vi "Untitled 4 (SubVI).vi"(10 "ID Query":string, 11 "VISA Refnum in":refnum<visa-resource-name>) -> (3 "read buffer":string)   [LabVIEW 2020]
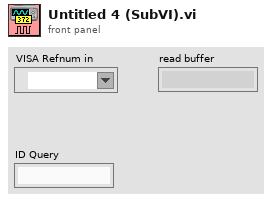
[diagram p1: front panel]
types:
  T1 = cluster{"Baud Rate":u32, "Parity":u16, "Data Bits":u16, "Stop Bits":u16, "Flow Control":u16}
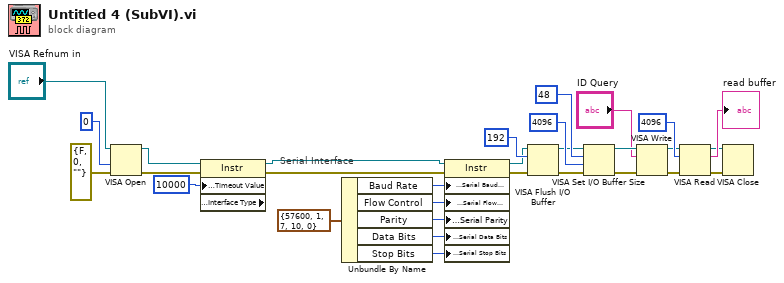
[diagram p0: block diagram]
diagram:
  # "Serial Interface"
  n1 = VISA Open(access mode=u32 0, error in (no error)=errorcluster {"status"=FALSE, "code"=0, "source"=""}, VISA resource name="VISA Refnum in") -> (VISA resource name=w5:refnum<visa-resource-name>, error out=w6:errorcluster)  [unwired: 2 in]
  n2 = property class="Instr" props=["General Settings:Timeout Value", "Interface Information:Interface Type"](reference=w5, error in=w6, "General Settings:Timeout Value"=u32 10000) -> (reference out=w7:refnum<visa-resource-name>, error out=w8:errorcluster)  [unwired: 1 out]
  n3 = Unbundle By Name(T1 {"Baud Rate"=57600, "Parity"=1, "Data Bits"=7, "Stop Bits"=10, "Flow Control"=0} ("Serial Configuration")) -> ("Baud Rate"=w20:u32, "Flow Control"=w24:u16, "Parity"=w22:u16, "Data Bits"=w21:u16, "Stop Bits"=w25:u16)
  n4 = property class="Instr"(reference=w7, error in=w8, "Serial Settings:Serial Baud Rate"=w20, "Serial Settings:Serial Flow Control"=w24, "Serial Settings:Serial Parity"=w22, "Serial Settings:Serial Data Bits"=w21, "Serial Settings:Serial Stop Bits"=w25) -> (reference out=w19:refnum<visa-resource-name>, error out=w17:errorcluster)
  n5 = VISA Flush I/O Buffer(VISA resource name=w19, mask (16)=u16 192, error in (no error)=w17) -> (VISA resource name out=w16:refnum<visa-resource-name>, error out=w18:errorcluster)
  n6 = VISA Set I/O Buffer Size(VISA resource name=w16, mask (16)=u16 48, size (4096)=u32 4096 ("size (0)"), error in (no error)=w18) -> (VISA resource name out=w30:refnum<visa-resource-name>, error out=w29:errorcluster)
  n7 = VISA Write(VISA resource name=w30, write buffer="ID Query", error in (no error)=w29) -> (VISA resource name out=w12:refnum<visa-resource-name>, error out=w11:errorcluster)  [unwired: 1 out]
  n8 = VISA Read(VISA resource name=w12, byte count=u32 4096, error in (no error)=w11) -> (VISA resource name out=w2:refnum<visa-resource-name>, read buffer=→"read buffer":string, error out=w1:errorcluster)  [unwired: 1 out]
  n9 = VISA Close(VISA resource name=w2, error in (no error)=w1) -> ()  [unwired: 1 out]
